vi "求水仙花数（2012）.vi"(1 "结束数":i32=999, 2 "开始数":i32=100) -> (0 "水仙花数":i32[](array[numeric]))   [LabVIEW 2012]
doc: "功能：\n\n求三位数中的水仙花数\n\n水仙花数的定义：\n\n所谓水仙花数，是指一个三位数，其各个位数的立方和等于该数本身，比如：\n\n153=1^3+5^+3^\n\ncsxcs_366创建"
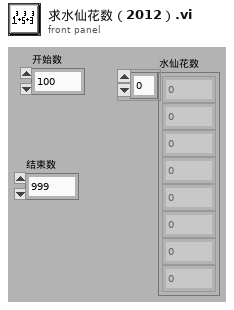
[diagram p1: front panel]
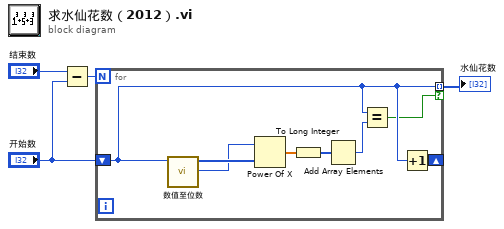
[diagram p0: block diagram]
diagram:
  n1 = Subtract(x="结束数", y="开始数") -> (x-y=w4:i32)
  n2 = for {
    N: w4 -> [_]
    shift-right: [w11] -> _
    shift-left: "开始数" -> [w6]
    tunnel: [w6] -> w1 mode=indexing if=w5
    n3 = call-poly "数值至位数.vi"("输入数值"=w6) -> ("总位数"=w7:i32, "位数数组"=w8:i32[])  [unwired: 8 in, 1 out]
    n4 = Power Of X(1:w8, 2:w7) -> (0:w10:dbl[])
    n5 = To Long Integer(number=w10) -> (32bit integer=w9:i32[])
    n6 = Add Array Elements(numeric array=w9) -> (sum=w12:i32)
    n7 = Equal?(x=w6, y=w12) -> (x = y?=w5:bool)
    n8 = Increment(x=w6) -> (x+1=w11:i32)
  }
  "水仙花数" <- w1
